vi "Untitled 1.vi"() -> ()   [LabVIEW 2009, in "Varian Magnet.lvclass"]
uses:
  Varian Magnet.lvclass
  <vilib>/DAQmx/create/channels.llb/DAQmx Create Channel (AO-Voltage-Basic).vi
  <vilib>/DAQmx/create/channels.llb/DAQmx Create Channel (AI-Voltage-Basic).vi
  <vilib>/DAQmx/write.llb/DAQmx Write (Analog DBL 1Chan 1Samp).vi
  <vilib>/DAQmx/read.llb/DAQmx Read (Analog DBL 1Chan 1Samp).vi
panel:
  in  "Amps Desired":dbl
  out "Waveform Chart":dbl(graph)
  out "Amps":dbl(knob) scale=0.0..1.0
  out "Raw voltage":dbl format="%0.4f"
  in  "stop":bool
  in  "data":dbl min=-9.0 max=9.0 format="%0.2f"
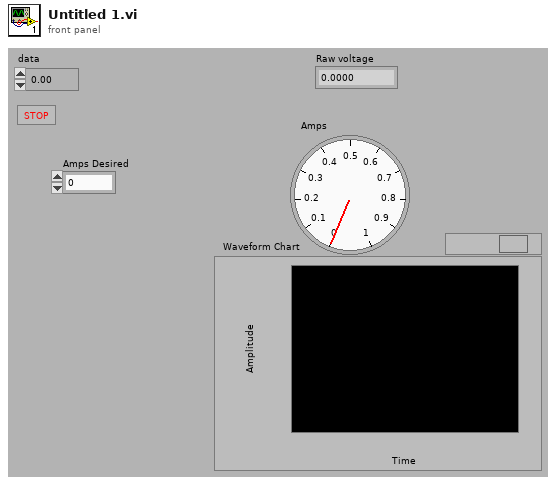
[diagram p1: front panel]
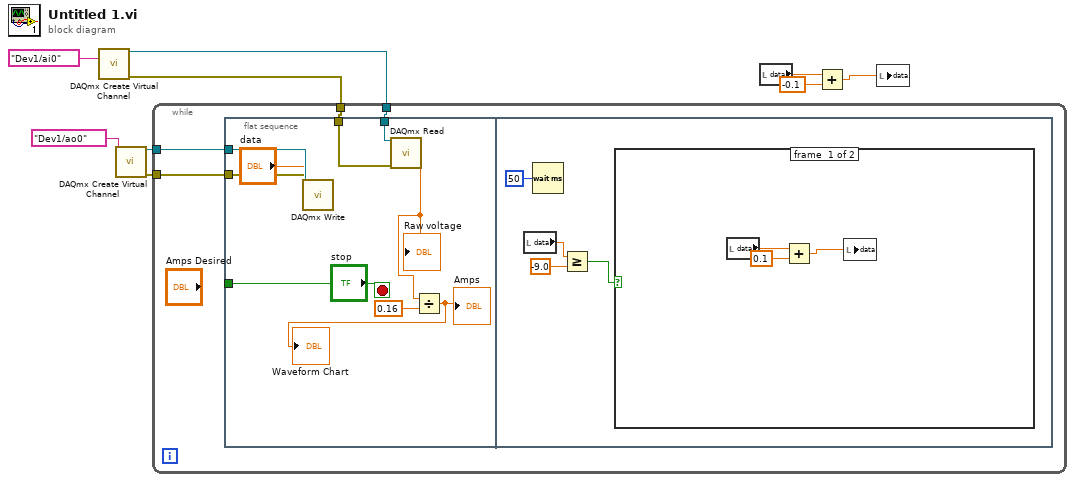
[diagram p0: block diagram]
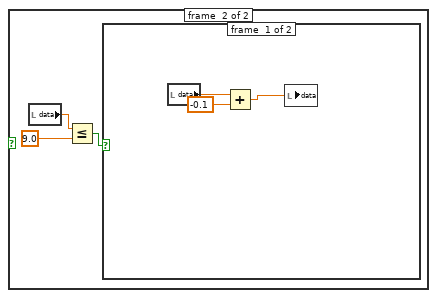
[diagram p2: hidden frame]
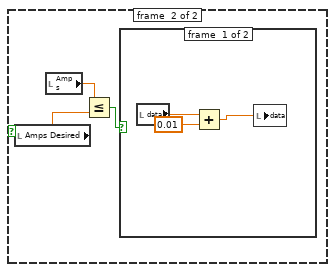
[diagram p3: hidden frame]
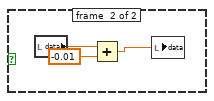
[diagram p4: hidden frame]
diagram:
  n1 = call-poly <vilib>:"DAQmx Create Virtual Channel.vi"("physical channels"=tag "Dev1/ai0") -> ("task out"=w6:refnum<k21>, "error out"=w5:errorcluster)  [unwired: 13 in]
  n2 = call-poly <vilib>:"DAQmx Create Virtual Channel.vi"("physical channels"=tag "Dev1/ao0") -> ("task out"=w8:refnum<k21>, "error out"=w7:errorcluster)  [unwired: 13 in]
  n3 = while {
    tunnel: w8 -> [w14]
    tunnel: w7 -> [w13]
    tunnel: w6 -> [w11]
    tunnel: w5 -> [w10]
    stop <- w12 stop-if-true
    n4 = flat-sequence {
      tunnel: w14 -> [w23]
      tunnel: w13 -> [w22]
      tunnel: ["stop"] -> w12
      tunnel: w11 -> [w19]
      tunnel: w10 -> [w18]
      frame #0 {
        n5 = call-poly <vilib>:"DAQmx Write.vi"("task/channels in"=w23, "data"="data", "error in"=w22) -> ()  [unwired: 10 in, 3 out]
        n6 = call-poly <vilib>:"DAQmx Read.vi"("task/channels in"=w19, "error in"=w18) -> ("data"=w16:dbl)  [unwired: 11 in, 2 out]
        "Raw voltage" <- w16
        n7 = Divide(x=w16, y=0.16) -> (x/y=→"Amps" →"Waveform Chart":dbl)
      }
      frame #1 {
        n8 = local read "data"() -> (w26:dbl)
        n9 = Wait (ms)(milliseconds to wait=u32 50) -> ()  [unwired: 1 out]
        n10 = Greater Or Equal?(x=w26, y=-9.0) -> (x >= y?=w25:bool)
        n11 = case shown="True" w25 {
          frame #0 {
            n12 = local read "data"() -> (w29:dbl)
            n13 = Add(x=w29, y=0.1) -> (x+y=w28:dbl)
            n14 = local write "data"(w28) -> ()
          }
          frame #1 {
            n15 = local read "data"() -> (w33:dbl)
            n16 = Less Or Equal?(x=w33, y=9.0) -> (x <= y?=w31:bool)
            n17 = case shown="True" w31 {
              frame #0 {
                n18 = local read "data"() -> (w35:dbl)
                n19 = Add(x=w35, y=-0.1) -> (x+y=w34:dbl)
                n20 = local write "data"(w34) -> ()
              }
              frame #1 {
                n21 = local read "Amps Desired"() -> (w37:dbl)
                n22 = local read "Amps"() -> (w38:dbl)
                n23 = Less Or Equal?(x=w38, y=w37) -> (x <= y?=w39:bool)
                n24 = case shown="False" w39 {
                  frame #0 {
                    n25 = local read "data"() -> (w41:dbl)
                    n26 = Add(x=w41, y=0.01) -> (x+y=w40:dbl)
                    n27 = local write "data"(w40) -> ()
                  }
                  frame #1 {
                    n28 = local read "data"() -> (w44:dbl)
                    n29 = Add(x=w44, y=-0.01) -> (x+y=w43:dbl)
                    n30 = local write "data"(w43) -> ()
                  }
                }
              }
            }
          }
        }
      }
    }
  }
  n31 = local read "data"() -> (w2:dbl)
  n32 = Add(x=w2, y=-0.1) -> (x+y=w3:dbl)
  n33 = local write "data"(w3) -> ()
